vi "myRIO__TCP_constants_byteRange__checkRange_All.vi"(11 "input_char":string) -> (3 "output_inRange":bool)   [LabVIEW 2014]
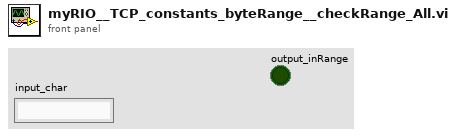
[diagram p1: front panel]
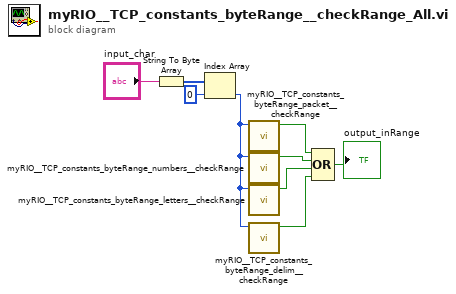
[diagram p0: block diagram]
diagram:
  n1 = String To Byte Array(string="input_char") -> (unsigned byte array=w8:u8[])
  n2 = Index Array(array=w8, index=0) -> (element=w2:u8)
  n3 = call "myRIO__TCP_constants_byteRange_packet__checkRange.vi"("input_byte"=w2) -> ("output_packet"=w6:bool)  [unwired: 8 in, 2 out]
  n4 = call "myRIO__TCP_constants_byteRange_numbers__checkRange.vi"("input_byte"=w2) -> ("output_numbers"=w5:bool)  [unwired: 8 in, 2 out]
  n5 = call "myRIO__TCP_constants_byteRange_letters__checkRange.vi"("input_byte"=w2) -> ("output_letters"=w4:bool)  [unwired: 8 in, 2 out]
  n6 = call "myRIO__TCP_constants_byteRange_delim__checkRange.vi"("input_byte"=w2) -> ("output_delim"=w1:bool)  [unwired: 9 in, 1 out]
  n7 = Compound Arithmetic op=OR(w6, w5, w4, w1) -> (→"output_inRange":bool)
